vi "Read Tactics.vi"(8 "error in (no error)":errorcluster, 11 "Role_v2 in":refnum<class "Role_v2.lvclass">) -> (0 "error out":errorcluster, 2 "Tactics":T1, 3 "Role_v2 out":refnum<class "Role_v2.lvclass">)   [LabVIEW 2023, in "Role_v2.lvclass"]
uses:
  Role_v2.lvclass
  TestTactic_class/TestTactic.lvclass
  Role_v2.lvclass/Role_v2.ctl
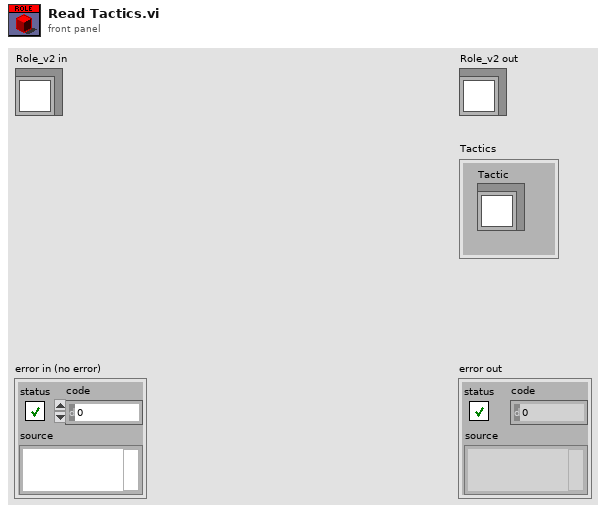
[diagram p1: front panel]
types:
  T1 = cluster{"Tactic":refnum<class "TestTactic.lvclass">}
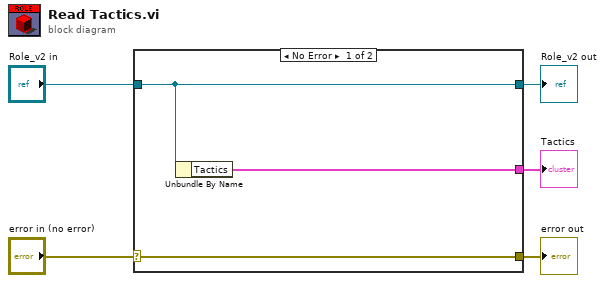
[diagram p0: block diagram]
diagram:
  n1 = case shown="No Error" "error in (no error)" {
    selector: "error in (no error)" -> [w8 w9]
    tunnel: [w8 w9] -> w4
    tunnel: [w7 w10] -> w2
    tunnel: "Role_v2 in" -> [w7 w10]
    tunnel: [w6 _] -> w1
    frame No Error {
      n2 = Unbundle By Name(w7) -> ("Tactics"=w6:T1)
    }
    frame Error {
    }
  }
  "error out" <- w4
  "Role_v2 out" <- w2
  "Tactics" <- w1
